vi "FitCol2Text.vi"(7 "Defer Updates?":bool=TRUE, 8 "error in (no error)":errorcluster, 9 "SetList Table ref":refnum<vi>, 10 "Col array":refnum<class "Column.lvclass">[](array[class]), 11 "Select Layout":i32(ring)=-1 items=["(On-the-fly)"=-2, "All"=-1, "pb only"=0, "selected"=1]) -> (0 "error out":errorcluster)   [LabVIEW 2013]
doc: "Temporarily resize visible columns so that all text in cells is visible."
uses:
  ColumnVIs/Column/Column.lvclass
  ColumnVIs/ModeCol/ModeCol.lvclass
  ColumnVIs/GroupCol/GroupCol.lvclass
  ColumnVIs/DigitalCol/DigitalCol.lvclass
  ColumnVIs/TriggerCol/TriggerCol.lvclass
  ColumnVIs/SingleValCol/SingleValCol.lvclass
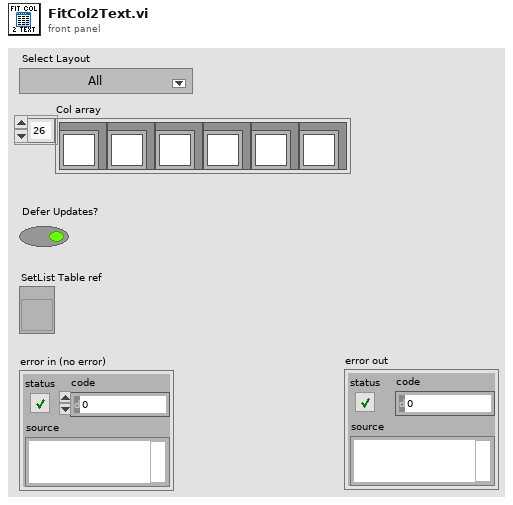
[diagram p1: front panel]
types:
  T1 = typedef "ColumnLayoutCluster.ctl" = cluster{"Label":string, "Color":u32, "Width":u32, "[disp?]":bool[]}
  T2 = cluster{"left":i16, "top":i16, "right":i16, "bottom":i16}
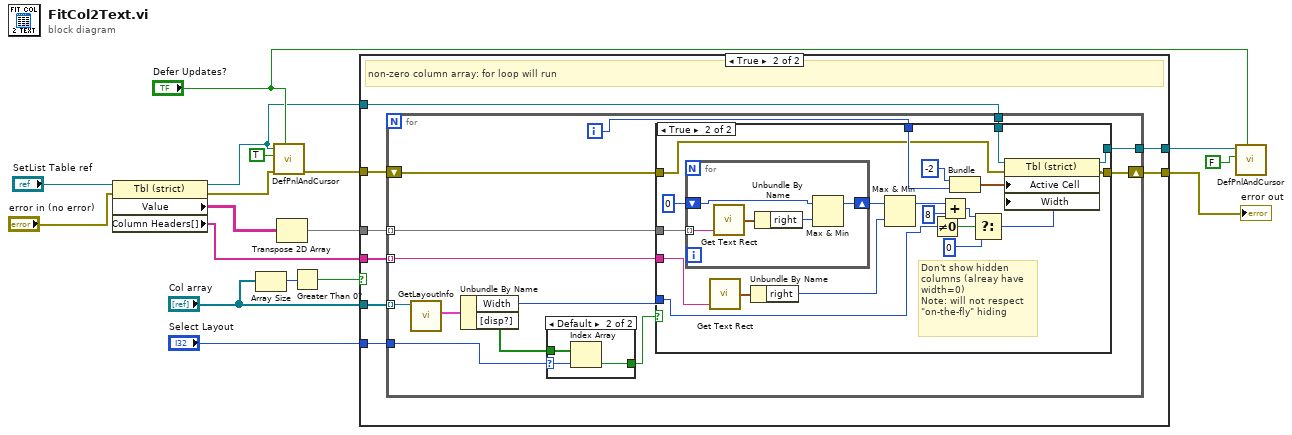
[diagram p0: block diagram]
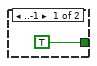
[diagram p3: hidden frame]
diagram:
  n1 = property class="Tbl (strict)"(reference="SetList Table ref", error in="error in (no error)") -> (reference out=w7:refnum<vi>, error out=w13:errorcluster, "Value"=w12:string[][], "Column Headers[]"=w11:string[])
  n2 = Array Size(array="Col array") -> (size(s)=w2:i32)
  n3 = call "DefPnlAndCursor.vi"("AllowDefPan? (T)"="Defer Updates?", "error in (no error)"=w13, "DeferPanUpdts?"=TRUE ("DeferPanUPdts?"), "Tbl Ctrl Refnum"=w7) -> ("error out"=w14:errorcluster)  [unwired: 7 in]
  n4 = Transpose 2D Array(2D array=w12) -> (transposed array=w17:string[][])
  n5 = Greater Than 0?(x=w2) -> (x > 0?=w1:bool)
  n6 = case shown="True" w1 {
    tunnel: w17 -> [_ w27]
    tunnel: w14 -> [w18 w26]
    tunnel: w11 -> [_ w25]
    tunnel: "Select Layout" -> [_ w24]
    tunnel: w7 -> [w19 w23]
    tunnel: [w18 w22] -> w5
    tunnel: [w19 w21] -> w4
    tunnel: "Col array" -> [_ w20]
    frame False {
      # "with zero columns, ensure Table ref exists so panel updates can be restored!"
    }
    frame True {
      # "non-zero column array: for loop will run"
      n7 = for {
        tunnel: w27 -> [w40] mode=indexing
        shift-right: [w37] -> w22
        shift-left: w26 -> [w38]
        tunnel: w25 -> [w36] mode=indexing
        tunnel: w20 -> [w35] mode=indexing
        tunnel: w24 -> [w30]
        tunnel: w23 -> [w29]
        tunnel: [w28] -> w21
        i -> [w39]
        n8 = call "GetLayoutInfo.vi"("Column in"=w35) -> ("Layout cluster"=w32:T1)  [unwired: 8 in, 2 out]
        n9 = Unbundle By Name(w32) -> ("Width"=w33:u32, "[disp?]"=w31:bool[])
        n10 = case shown="Default" w30 {
          selector: w30 -> [_ w42]
          tunnel: [TRUE ("Displayed?") w44] -> w34
          tunnel: w31 -> [_ w43]
          frame ..-1 {
          }
          frame Default {
            n11 = Index Array(array=w43, index=w42) -> (element=w44:bool)
          }
        }
        n12 = case shown="True" w34 {
          tunnel: w40 -> [_ w64]
          tunnel: w39 -> [_ w62]
          tunnel: w38 -> [w46 w55]
          tunnel: [w46 w60] -> w37
          tunnel: w36 -> [_ w56]
          tunnel: w33 -> [_ w49]
          tunnel: w29 -> [w45 w48]
          tunnel: [w45 w47] -> w28
          frame False {
          }
          frame True {
            # "Don't show hidden\ncolumns (alreay have\nwidth=0)\nNote: will not respect \n\"on-the-fly\" hiding"
            n13 = for {
              shift-right: [w68] -> w59
              shift-left: 0 -> [w70]
              tunnel: w64 -> [w67] mode=indexing
              n14 = call <vilib>:"Get Text Rect.vi"("text"=w67) -> ("rect"=w71:T2)  [unwired: 8 in]
              n15 = Unbundle By Name(w71) -> ("right"=w69:i16)
              n16 = Max & Min(x=w70, y=w69) -> (max(x,y)=w68:i32)  [unwired: 1 out]
            }
            n17 = call <vilib>:"Get Text Rect.vi"("text"=w56) -> ("rect"=w58:T2)  [unwired: 8 in]
            n18 = Unbundle By Name(w58) -> ("right"=w57:i16)
            n19 = Max & Min(x=w59, y=w57) -> (max(x,y)=w52:i32)  [unwired: 1 out]
            n20 = Not Equal To 0?(x=w49) -> (x != 0?=w51:bool)
            n21 = Add(x=w52, y=8) -> (x+y=w54:i32)
            n22 = Bundle("Row"=-2, w62) -> (w61:cluster{"Row":i32, i32})  [unwired: 1 in]
            n23 = Select(t=w54, s=w51, f=0 ("y")) -> (s? t:f=w53:i32)
            n24 = property on="Property Node" class="Tbl (strict)"(reference=w48, error in=w55, "Active Cell"=w61, "Width"=w53) -> (reference out=w47:refnum<vi>, error out=w60:errorcluster)
          }
        }
      }
    }
  }
  "error out" <- w5
  n25 = call "DefPnlAndCursor.vi"("AllowDefPan? (T)"="Defer Updates?", "DeferPanUpdts?"=FALSE ("DeferPanUPdts?"), "Tbl Ctrl Refnum"=w4) -> ()  [unwired: 8 in, 1 out]
